vi "一体站流程自动启动.vi"(10 "二级进样":bool, 11 "参数":T1) -> ()   [LabVIEW 2016, in "PLC.lvlib"]
uses:
  PLC.lvlib
panel:
  out "s? t:f":enum16{"初始化", "采配水启动", "仪器操作", "反冲洗", "结束"}(ring)
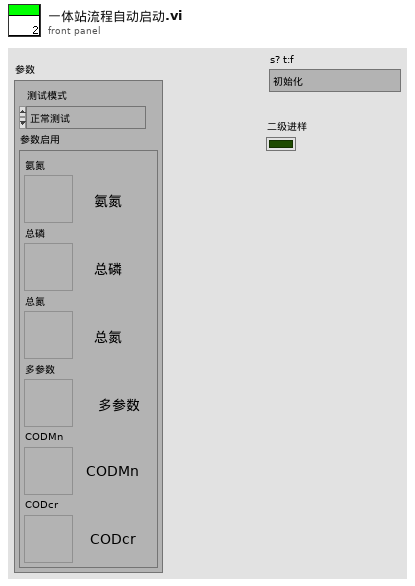
[diagram p1: front panel]
types:
  T1 = cluster{"测试模式":enum16{"正常测试", "集成干预"}, "参数启用":cluster{"氨氮":bool, "总磷":bool, "总氮":bool, "多参数":bool, "CODMn":bool, "CODcr":bool}}
  T2 = cluster{"命令":string, cluster{"starting address":u16, "holding register value":u16}}
  T3 = enum16{"启动测量", "标样核查", "零点核查", "跨度核查", "空白测试", "平行样测试", "加标回收", "空白校准", "标样校准", "初始化（清洗）", "停止测试", "仪器重启", "校时", "模式设置", "测量间隔设置"}
  T4 = cluster{"时间标识":timestamp, "设备":string, "日志信息":string, "流程参数":string}
  T5 = cluster{"测量模式":enum16{"水样测量", "标样核查", "零点核查", "跨度核查", "空白测试", "加标回收", "平行样", "校零", "校标"}}
  T6 = cluster{"时间标识":timestamp, "设备":string, "日志信息":string}
  T7 = enum16{"空闲", "水样测试", "标样核查", "零点核查", "跨度核查", "空白测试", "平行样测试", "加标回收", "空白校准", "标样校准", "初始化（清洗）"}
  T8 = cluster{"R0":i16, "R1":i16, "R2":i16, "R3":i16, "R4":i16, "R5":i16, "R6":i16, "R7":i16, "R8":i16, "R9":i16, "R10":i16, "R11":i16, "R12":i16, "R13":i16, "R14":i16, "R15":i16, "R16":i16, "R17":i16, "R18":i16, "R19":i16, "R20":i16, "R21":i16, "R22":i16, "R23":i16, "R24":i16, "R25":i16, "R26":i16, "R27":i16, "R28":i16, "R29":i16, "R30":i16, "R31":i16, "R32":i16, "R33":i16, "R34":i16, "R35":i16, "R36":i16, "R37":i16, "R38":i16, "R39":i16, "R40":i16, "R41":i16, "R42":i16, "R43":i16, "R44":i16, "R45":i16, "R46":i16, "R47":i16, "R48":i16, "R49":i16, "R50":i16, "R51":i16, "R52":i16, "R53":i16, "R54":i16, "R55":i16, "R56":i16}
  T9 = cluster{"R100":i16, "R101":i16, "R102":i16, "R103":i16, "R104":i16, "R105":i16, "R106":i16, "R107":i16, "R108":i16, "R109":i16, "R110":i16, "R111":i16, "R112":i16, "R113":i16, "R114":i16, "R115":i16, "R116":i16, "R117":i16, "R118":i16, "R119":i16, "R120":i16, "R121":i16, "R122":i16, "R123":i16}
  T10 = enum32{"Bad", "Idle", "Run top level", "Running"}
  T11 = cluster{"氨氮":bool, "总磷":bool, "总氮":bool, "多参数":bool, "CODMn":bool, "CODcr":bool}
  T12 = cluster{"时间标识":timestamp, "参数":string, "集成干预测试浓度值":dbl, "集成干预前测试时间":timestamp, "集成干预前测试浓度值":dbl}
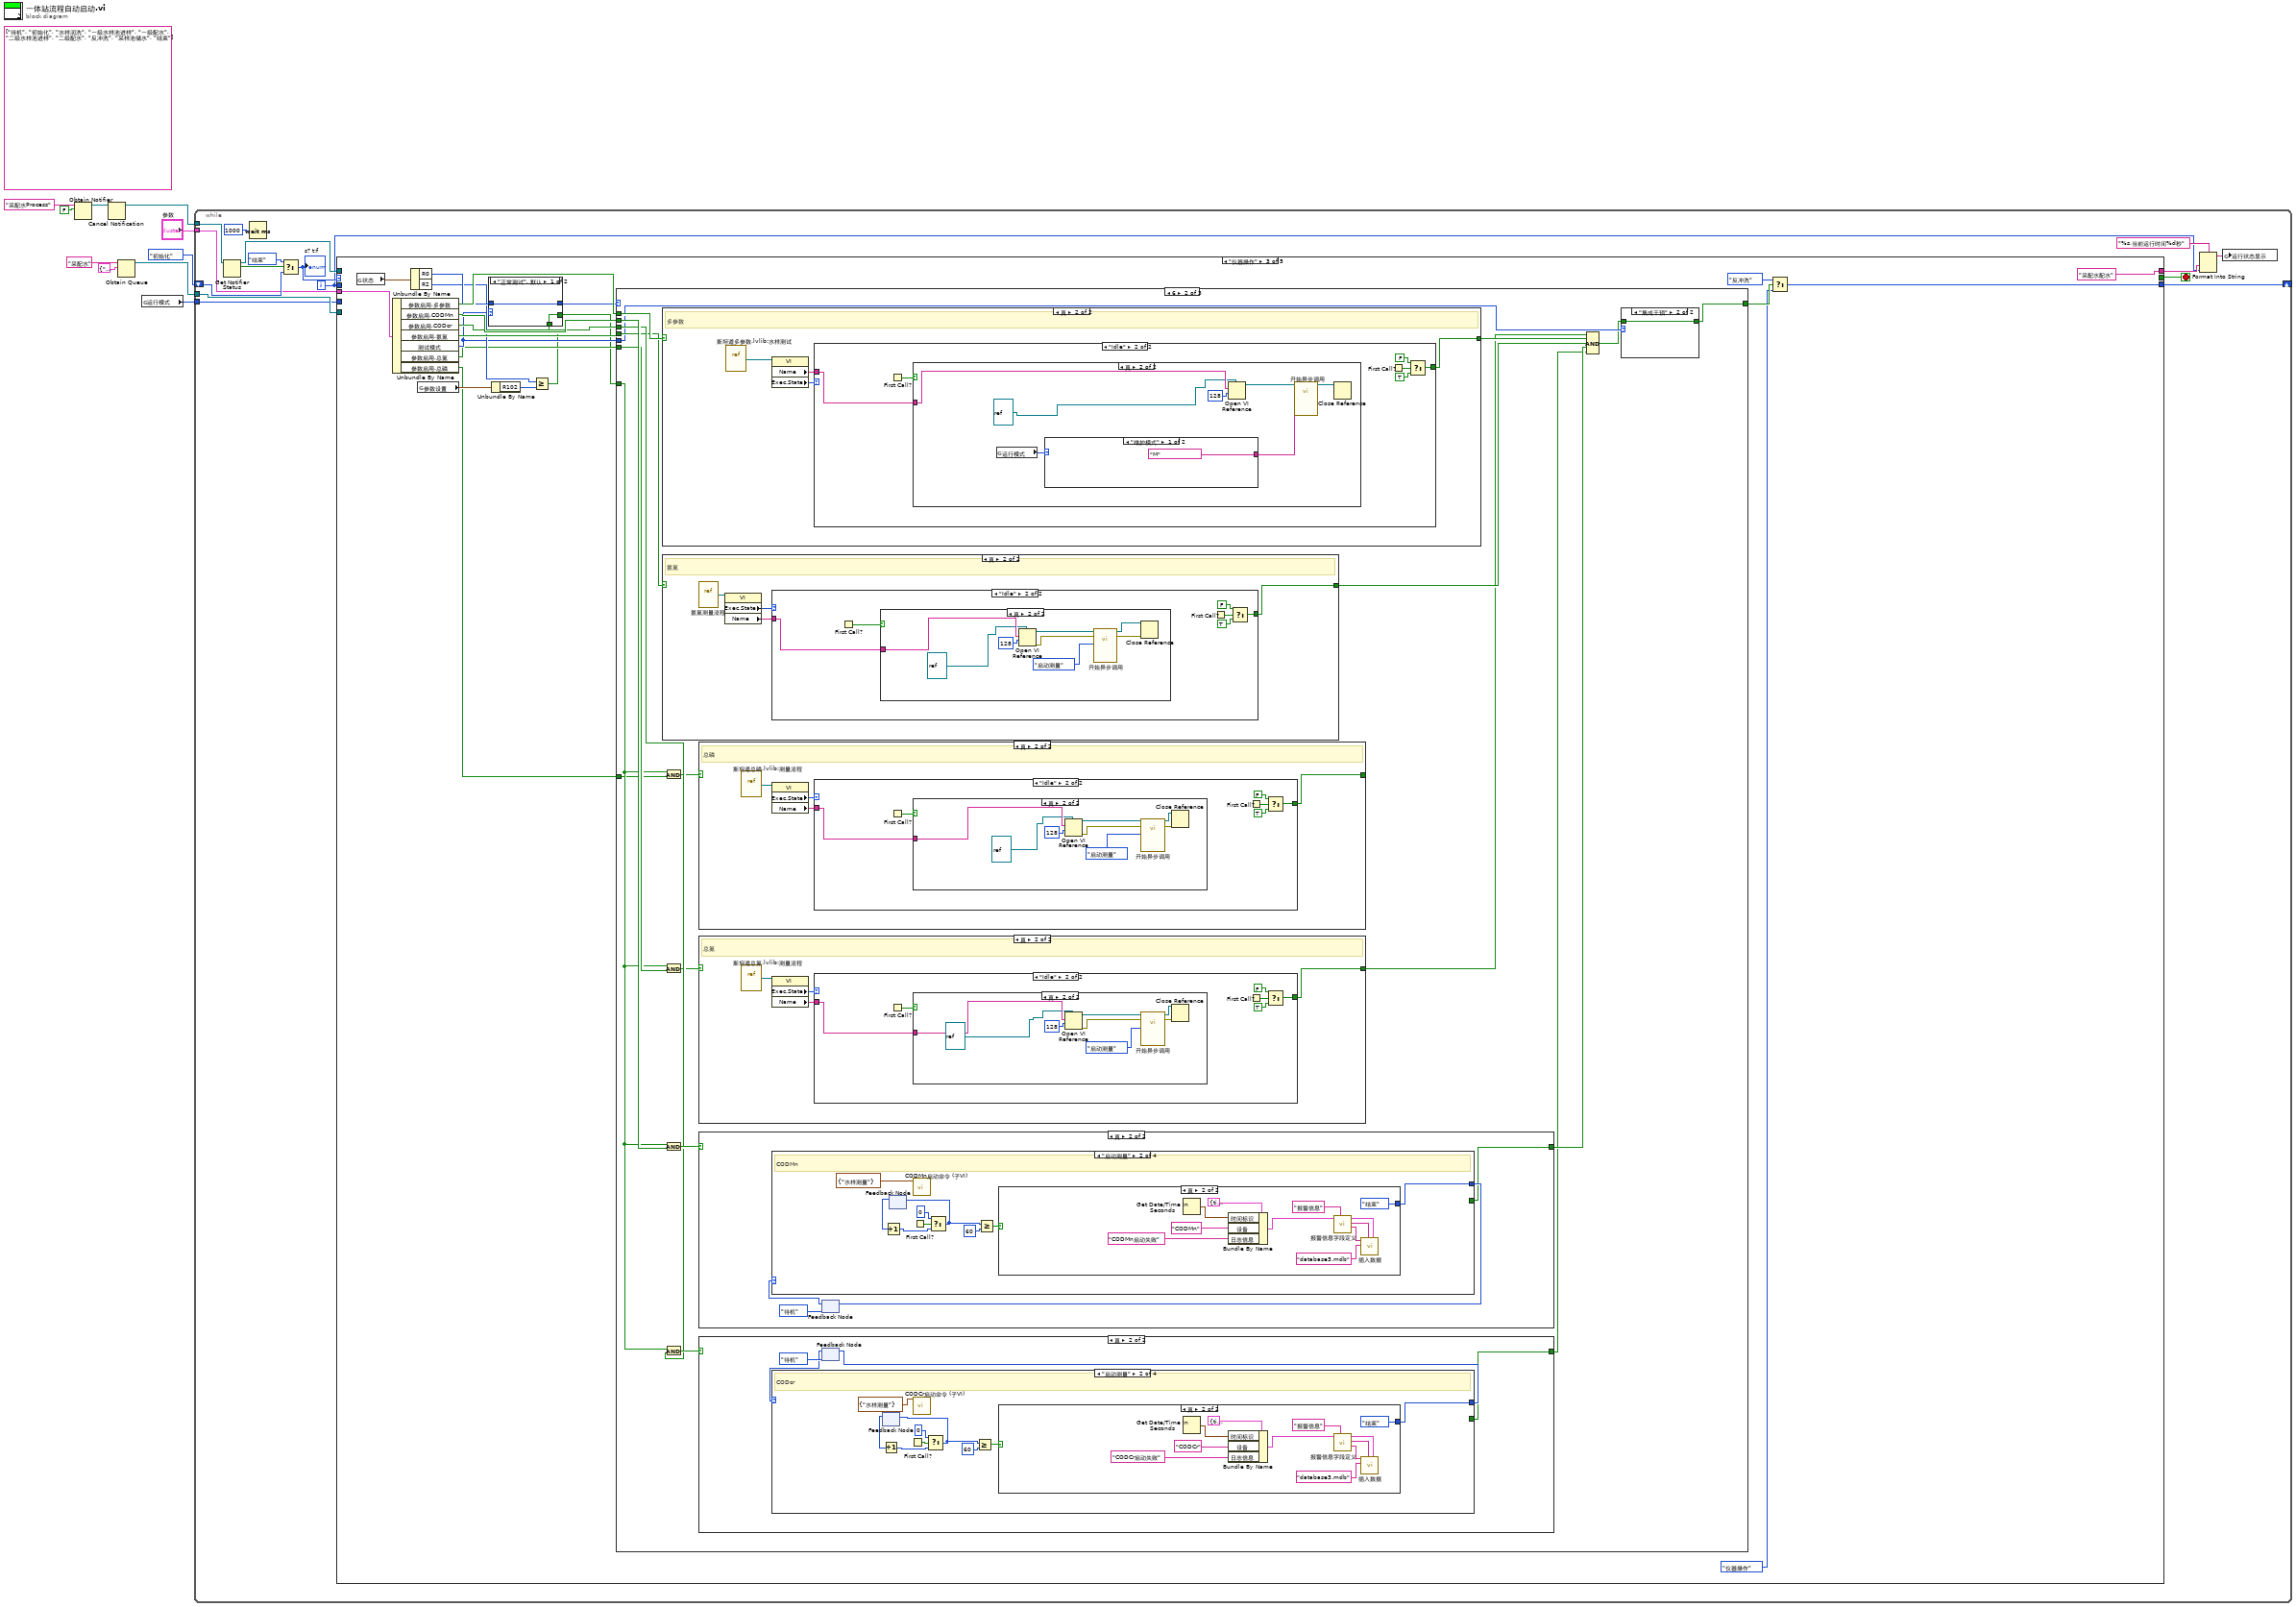
[diagram p0: block diagram]
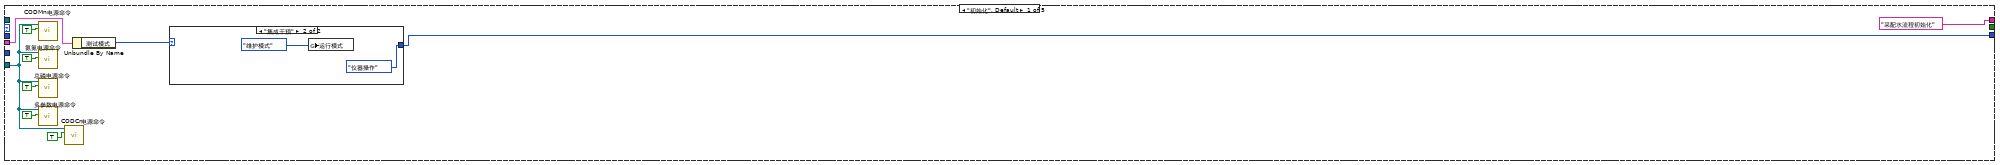
[diagram p2: hidden frame]
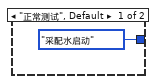
[diagram p3: hidden frame]
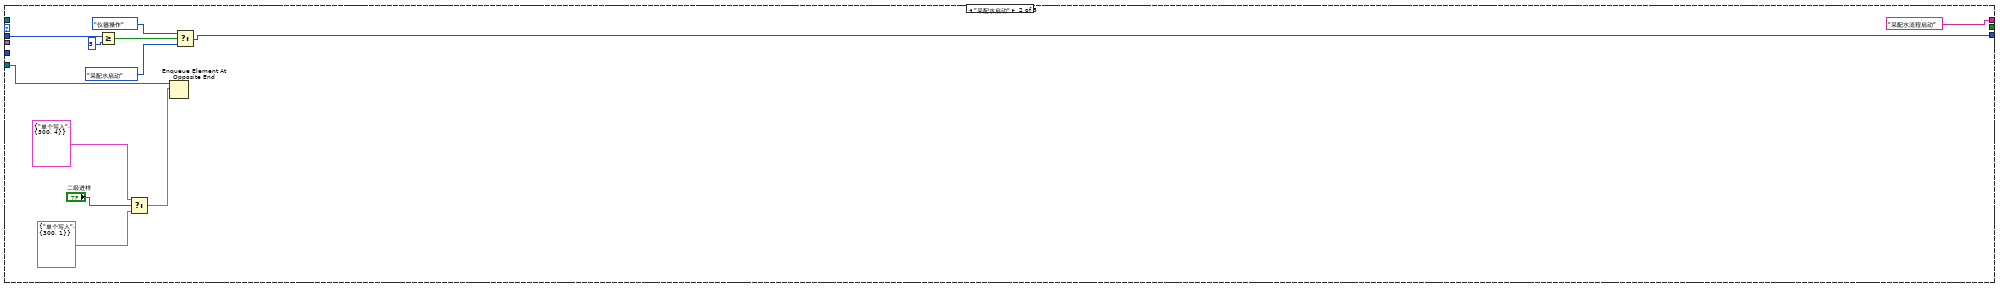
[diagram p4: hidden frame]
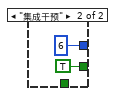
[diagram p5: hidden frame]
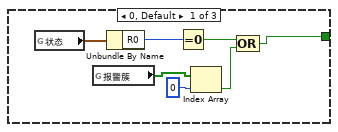
[diagram p6: hidden frame]
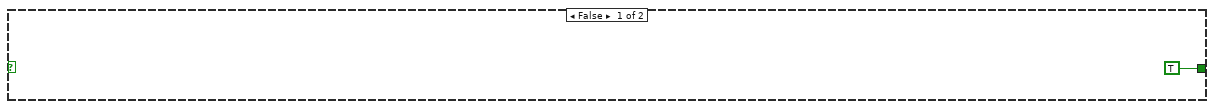
[diagram p7: hidden frame]
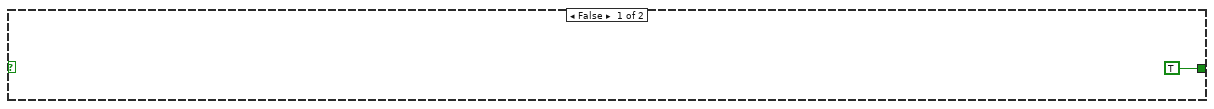
[diagram p10: hidden frame]
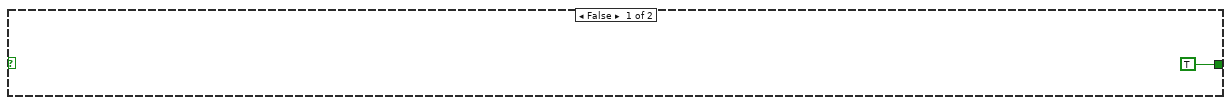
[diagram p14: hidden frame]
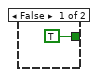
[diagram p17: hidden frame]
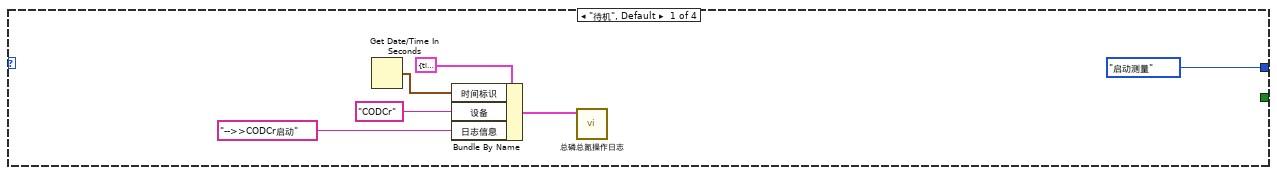
[diagram p18: hidden frame]
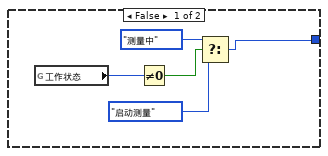
[diagram p19: hidden frame]
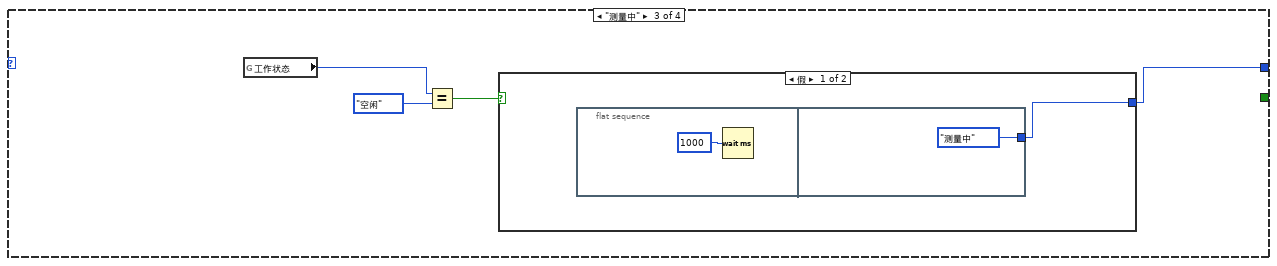
[diagram p20: hidden frame]
diagram:
  (unwired) string[][] [["待机"], ["初始化"], ["水样润洗"], ["一级水样池进样"], ["一级配水"], ["二级水样池进样"], ["二级配水"], ["反冲洗"], ["采样池储水"], ["结束"]] ("项名")
  n1 = Obtain Notifier(name (unnamed)="采配水Process" ("名称（未命名）"), notification data type=FALSE) -> (notifier out=w4:refnum<notifier>)  [unwired: 2 in, 2 out]
  n2 = Cancel Notification(0:w4) -> (8:w3:refnum<notifier>)  [unwired: 1 in, 2 out]
  n3 = Obtain Queue(name (unnamed)="采配水" ("名称（未命名）"), element data type=cluster{"命令":string, "数据":variant} {"命令"="", "数据"=variant}) -> (queue out=w7:refnum<queue>)  [unwired: 3 in, 2 out]
  n4 = global read "系统设置全局变量.vi" "运行模式"() -> (w1:enum16{"维护模式", "常规模式", "应急模式", "质控模式"})
  n5 = while {
    shift-right: [w23] -> _
    shift-left: enum16{"初始化", "采配水启动", "仪器操作", "反冲洗", "结束"}."初始化" ("枚举") -> [w19]
    tunnel: w7 -> [w26]
    tunnel: w3 -> [w22]
    tunnel: "参数" -> [w13]
    tunnel: w1 -> [w12]
    i -> [w11]
    stop <- w25 stop-if-true
    n6 = Get Notifier Status(notifier=w22) -> (notifier out=w14:refnum<notifier>, current notification=w21:bool)  [unwired: 1 in, 3 out]
    n7 = Wait (ms)(milliseconds to wait=u32 1000 ("等待时间（毫秒）")) -> ()  [unwired: 1 out]
    n8 = Select(t=enum16{"初始化", "采配水启动", "仪器操作", "反冲洗", "结束"}."结束" ("枚举"), s=w21, f=w19) -> (s? t:f=w18:enum16{"初始化", "采配水启动", "仪器操作", "反冲洗", "结束"})
    "s? t:f" <- w18
    n9 = case shown="\"仪器操作\"" w18 {
      tunnel: w26 -> [w31 w51 _ _ w456]
      tunnel: [_ _ _ _ TRUE] -> w25
      tunnel: [w30 w44 w67 w288 enum16{"初始化", "采配水启动", "仪器操作", "反冲洗", "结束"}."结束" ("枚举")] -> w23
      tunnel: ["采配水流程初始化" "采配水流程启动" "采配水配水" "等待测试完成" "采配水结束"] -> w15
      tunnel: w14 -> [_ _ _ _ w457]
      tunnel: w13 -> [w28 _ w70 w287 w453]
      tunnel: w12 -> [_ _ _ _ w452]
      tunnel: w11 -> [_ w49 _ _ _]
      frame "初始化", Default {
        n10 = call "CODMn电源命令.vi"("通电/断电"=TRUE, "队列"=w31) -> ()  [unwired: 9 in, 1 out]
        n11 = call "氨氮电源命令.vi"("通电/断电"=TRUE, "队列"=w31) -> ()  [unwired: 9 in, 1 out]
        n12 = call "总磷电源命令.vi"("通电/断电"=TRUE, "队列"=w31) -> ()  [unwired: 9 in, 1 out]
        n13 = call "多参数电源命令.vi"("通电/断电"=TRUE, "队列"=w31) -> ()  [unwired: 9 in, 1 out]
        n14 = call "CODCr电源命令.vi"("通电/断电"=TRUE, "队列"=w31) -> ()  [unwired: 9 in, 1 out]
        n15 = Unbundle By Name(w28) -> ("测试模式"=w27:enum16{"正常测试", "集成干预"})
        n16 = case shown="\"集成干预\"" w27 {
          tunnel: [enum16{"初始化", "采配水启动", "仪器操作", "反冲洗", "结束"}."采配水启动" ("枚举") enum16{"初始化", "采配水启动", "仪器操作", "反冲洗", "结束"}."仪器操作" ("枚举")] -> w30
          frame "正常测试", Default {
          }
          frame "集成干预" {
            n17 = global write "系统设置全局变量.vi" "运行模式"(enum16{"维护模式", "常规模式", "应急模式", "质控模式"}."维护模式" ("运行模式")) -> ()
          }
        }
      }
      frame "采配水启动" {
        n18 = Greater Or Equal?(x=w49, y=5) -> (x >= y?=w47:bool)
        n19 = Select(t=T2 {"命令"="单个写入", {"starting address"=300, "holding register value"=4}} ("元素"), s="二级进样", f=T2 {"命令"="单个写入", {"starting address"=300, "holding register value"=1}} ("元素")) -> (s? t:f=w40:T2)
        n20 = Enqueue Element At Opposite End(queue=w51, element=w40) -> ()  [unwired: 2 in, 3 out]
        n21 = Select(t=enum16{"初始化", "采配水启动", "仪器操作", "反冲洗", "结束"}."仪器操作" ("枚举"), s=w47, f=enum16{"初始化", "采配水启动", "仪器操作", "反冲洗", "结束"}."采配水启动" ("枚举")) -> (s? t:f=w44:enum16{"初始化", "采配水启动", "仪器操作", "反冲洗", "结束"})
      }
      frame "仪器操作" {
        n22 = global read "采配水全局变量.vi" "状态"() -> (w72:T8)
        n23 = Unbundle By Name(w70) -> ("参数启用.多参数"=w65:bool, "参数启用.CODMn"=w64:bool, "参数启用.CODcr"=w63:bool, "参数启用.氨氮"=w62:bool, "测试模式"=w56:enum16{"正常测试", "集成干预"}, "参数启用.总氮"=w55:bool, "参数启用.总磷"=w54:bool)
        n24 = Unbundle By Name(w72) -> ("R0"=w61:i16, "R2"=w57:i16)
        n25 = global read "采配水全局变量.vi" "参数设置"() -> (w58:T9)
        n26 = Unbundle By Name(w58) -> ("R102"=w59:i16)
        n27 = Greater Or Equal?(x=w57, y=w59) -> (x >= y?=w53:bool)
        n28 = case shown="\"正常测试\", 默认" w56 {
          tunnel: w61 -> [w74 _]
          tunnel: [w74 i16 6 ("R0")] -> w60
          tunnel: w53 -> [w73 _]
          tunnel: [w73 TRUE] -> w52
          frame "正常测试", Default {
          }
          frame "集成干预" {
          }
        }
        n29 = case shown="6" w60 {
          tunnel: [w78 w90 TRUE] -> w69
          tunnel: w65 -> [_ w102 _]
          tunnel: w64 -> [_ w101 _]
          tunnel: w63 -> [_ w98 _]
          tunnel: w62 -> [_ w97 _]
          tunnel: w52 -> [_ w86 _]
          tunnel: w56 -> [_ w92 _]
          tunnel: w55 -> [_ w89 _]
          tunnel: w54 -> [_ w85 _]
          frame 0, Default {
            n30 = global read "采配水全局变量.vi" "状态"() -> (w81:T8)
            n31 = global read "采配水全局变量.vi" "报警簇"() -> (w82:bool[])
            n32 = Unbundle By Name(w81) -> ("R0"=w80:i16)
            n33 = Equal To 0?(x=w80) -> (x = 0?=w83:bool)
            n34 = Index Array(array=w82, index=0 ("索引")) -> (element=w77:bool)
            n35 = Compound Arithmetic op=OR ("复合运算")(w83, w77) -> (w78:bool)
          }
          frame 6 {
            n36 = case shown="真" w102 {
              tunnel: [TRUE ("t") w268] -> w96
              frame False {
              }
              frame True {
                # "多参数"
                n37 = vi-ref "斯坦道多参数.lvlib:水样测试.vi"() -> (w266:refnum<vi>)
                n38 = property class="VI"(reference=w266) -> ("Name"=w265:string, "Exec.State"=w267:T10)  [unwired: 1 in, 2 out]
                n39 = case shown="\"Idle\"" w267 {
                  tunnel: w265 -> [_ w274]
                  tunnel: [_ w269] -> w268
                  frame "Bad", Default {
                  }
                  frame "Idle" {
                    n40 = First Call?() -> (First Call?: T/F=w273:bool)
                    n41 = case shown="真" w273 {
                      tunnel: w274 -> [_ w280]
                      frame False {
                      }
                      frame True {
                        n42 = global read "系统设置全局变量.vi" "运行模式"() -> (w277:enum16{"维护模式", "常规模式", "应急模式", "质控模式"})
                        n43 = case shown="\"维护模式\"" w277 {
                          tunnel: ["M" ("数据标记表") "N" ("数据标记表")] -> w276
                          frame "维护模式" {
                          }
                          frame "常规模式", Default {
                          }
                        }
                        n44 = Open VI Reference(type specifier VI Refnum (for type only)=refnum<vi> refnum, vi path=w280, options=128 ("选项")) -> (vi reference=w279:refnum<vi>)  [unwired: 3 in, 1 out]
                        n45 = call-by-ref "开始异步调用"(reference=w279, "数据标记表"=w276) -> (reference out=w278:refnum<vi>)  [unwired: 12 in, 1 out]
                        n46 = Close Reference(reference=w278) -> ()  [unwired: 1 in, 1 out]
                      }
                    }
                    n47 = First Call?() -> (First Call?: T/F=w272:bool)
                    n48 = Select(t=FALSE, s=w272, f=TRUE) -> (s? t:f=w269:bool)
                  }
                }
              }
            }
            n49 = case "条件结构" shown="真" w97 {
              tunnel: [TRUE ("t") w143] -> w95
              frame False {
              }
              frame True {
                # "氨氮"
                n50 = vi-ref "氨氮测量流程.vi"() -> (w146:refnum<vi>)
                n51 = property class="VI"(reference=w146) -> ("Exec.State"=w145:T10, "Name"=w144:string)  [unwired: 1 in, 2 out]
                n52 = case shown="\"Idle\"" w145 {
                  tunnel: w144 -> [_ w152]
                  tunnel: [_ w147] -> w143
                  frame "Bad", Default {
                  }
                  frame "Idle" {
                    n53 = First Call?() -> (First Call?: T/F=w151:bool)
                    n54 = case shown="真" w151 {
                      tunnel: w152 -> [_ w157]
                      frame False {
                      }
                      frame True {
                        n55 = Open VI Reference(type specifier VI Refnum (for type only)=refnum<vi> refnum, vi path=w157, options=128 ("选项")) -> (vi reference=w155:refnum<vi>, error out=w158:errorcluster)  [unwired: 3 in]
                        n56 = call-by-ref "开始异步调用"(reference=w155, error in=w158, "控制命令"=T3."启动测量") -> (reference out=w159:refnum<vi>, error out=w160:errorcluster)  [unwired: 11 in]
                        n57 = Close Reference(reference=w159, error in (no error)=w160) -> ()  [unwired: 1 out]
                      }
                    }
                    n58 = First Call?() -> (First Call?: T/F=w150:bool)
                    n59 = Select(t=FALSE, s=w150, f=TRUE) -> (s? t:f=w147:bool)
                  }
                }
              }
            }
            n60 = And(x=w86, y=w85) -> (x .and. y?=w84:bool)
            n61 = And(x=w86, y=w89) -> (x .and. y?=w88:bool)
            n62 = And(x=w86, y=w101) -> (x .and. y?=w100:bool)
            n63 = And(x=w86, y=w98) -> (x .and. y?=w99:bool)
            n64 = case "条件结构" shown="真" w84 {
              tunnel: [TRUE ("t") w104] -> _
              frame False {
              }
              frame True {
                # "总磷"
                n65 = vi-ref "斯坦道总磷.lvlib:测量流程.vi"() -> (w107:refnum<vi>)
                n66 = property class="VI"(reference=w107) -> ("Exec.State"=w106:T10, "Name"=w105:string)  [unwired: 1 in, 2 out]
                n67 = case shown="\"Idle\"" w106 {
                  tunnel: w105 -> [_ w113]
                  tunnel: [_ w108] -> w104
                  frame "Bad", Default {
                  }
                  frame "Idle" {
                    n68 = First Call?() -> (First Call?: T/F=w112:bool)
                    n69 = case shown="真" w112 {
                      tunnel: w113 -> [_ w118]
                      frame False {
                      }
                      frame True {
                        n70 = Open VI Reference(type specifier VI Refnum (for type only)=refnum<vi> refnum, vi path=w118, options=128 ("选项")) -> (vi reference=w116:refnum<vi>, error out=w119:errorcluster)  [unwired: 3 in]
                        n71 = call-by-ref "开始异步调用"(reference=w116, error in=w119, "控制命令"=T3."启动测量") -> (reference out=w120:refnum<vi>, error out=w121:errorcluster)  [unwired: 11 in]
                        n72 = Close Reference(reference=w120, error in (no error)=w121) -> ()  [unwired: 1 out]
                      }
                    }
                    n73 = First Call?() -> (First Call?: T/F=w111:bool)
                    n74 = Select(t=FALSE, s=w111, f=TRUE) -> (s? t:f=w108:bool)
                  }
                }
              }
            }
            n75 = case "条件结构" shown="真" w88 {
              tunnel: [TRUE ("t") w123] -> w87
              frame False {
              }
              frame True {
                # "总氮"
                n76 = vi-ref "斯坦道总氮.lvlib:测量流程.vi"() -> (w126:refnum<vi>)
                n77 = property class="VI"(reference=w126) -> ("Exec.State"=w125:T10, "Name"=w124:string)  [unwired: 1 in, 2 out]
                n78 = case shown="\"Idle\"" w125 {
                  tunnel: w124 -> [_ w132]
                  tunnel: [_ w127] -> w123
                  frame "Bad", Default {
                  }
                  frame "Idle" {
                    n79 = First Call?() -> (First Call?: T/F=w131:bool)
                    n80 = case shown="真" w131 {
                      tunnel: w132 -> [_ w137]
                      frame False {
                      }
                      frame True {
                        n81 = Open VI Reference(type specifier VI Refnum (for type only)=refnum<vi> refnum, vi path=w137, options=128 ("选项")) -> (vi reference=w135:refnum<vi>, error out=w138:errorcluster)  [unwired: 3 in]
                        n82 = call-by-ref "开始异步调用"(reference=w135, error in=w138, "控制命令"=T3."启动测量") -> (reference out=w139:refnum<vi>, error out=w140:errorcluster)  [unwired: 11 in]
                        n83 = Close Reference(reference=w139, error in (no error)=w140) -> ()  [unwired: 1 out]
                      }
                    }
                    n84 = First Call?() -> (First Call?: T/F=w130:bool)
                    n85 = Select(t=FALSE, s=w130, f=TRUE) -> (s? t:f=w127:bool)
                  }
                }
              }
            }
            n86 = case shown="真" w100 {
              tunnel: [TRUE w214] -> w94
              frame False {
              }
              frame True {
                n87 = feedback #1(enum16{"待机", "启动测量", "测量中", "结束"}."待机") -> (w216:enum16{"待机", "启动测量", "测量中", "结束"})
                n88 = case shown="\"启动测量\"" w216 {
                  tunnel: [enum16{"待机", "启动测量", "测量中", "结束"}."启动测量" w232 w251 enum16{"待机", "启动测量", "测量中", "结束"}."结束"] -> w215
                  tunnel: [_ _ _ TRUE] -> w214
                  frame "待机", Default {
                    n89 = Get Date/Time In Seconds() -> (seconds since 1Jan1904=w222:timestamp)
                    n90 = Bundle By Name(cluster=T4 {"时间标识"=timestamp(0 s since 1904-01-01), "设备"="", "日志信息"="", "流程参数"=""} ("data in"), "时间标识"=w222, "设备"="CODMn", "日志信息"="-->>CODMn启动") -> (w218:T4)
                    n91 = call "总磷总氮操作日志.vi"("data in"=w218) -> ()  [unwired: 11 in]
                  }
                  frame "启动测量" {
                    # "CODMn"
                    n92 = feedback #2() -> (w228:i32)  [unwired: 1 in]
                    n93 = Increment(x=w228) -> (x+1=w229:i32)
                    n94 = First Call?() -> (First Call?: T/F=w227:bool)
                    n95 = call "CODMn启动命令 (子VI).vi"("启动测量模式"=T5 {"测量模式"=enum."水样测量"}) -> ()  [unwired: 11 in]
                    n96 = Select(t=0, s=w227, f=w229) -> (s? t:f=w230:i32)
                    n97 = feedback-in #2(w230) -> ()
                    n98 = Greater Or Equal?(x=w230, y=60) -> (x >= y?=w225:bool)
                    n99 = case shown="真" w225 {
                      tunnel: [w234 enum16{"待机", "启动测量", "测量中", "结束"}."结束"] -> w232
                      frame False {
                        n100 = global read "运行时序全局变量.vi" "多列列表框"() -> (w233:i32)
                        n101 = Not Equal To 0?(x=w233) -> (x != 0?=w235:bool)
                        n102 = Select(t=enum16{"待机", "启动测量", "测量中", "结束"}."测量中", s=w235, f=enum16{"待机", "启动测量", "测量中", "结束"}."启动测量") -> (s? t:f=w234:enum16{"待机", "启动测量", "测量中", "结束"})
                      }
                      frame True {
                        n103 = Get Date/Time In Seconds() -> (seconds since 1Jan1904=w244:timestamp)
                        n104 = Bundle By Name(cluster=T6 {"时间标识"=timestamp(0 s since 1904-01-01), "设备"="", "日志信息"=""} ("data in"), "时间标识"=w244, "设备"="CODMn", "日志信息"="CODMn启动失败") -> (w238:T6)
                        n105 = call "报警信息字段定义.vi"("table输入"="报警信息", "data in"=w238) -> ("table输出"=w241:string, "columns"=w242:string[], "data out"=w243:T6)  [unwired: 7 in]
                        n106 = call "插入数据.vi"("data"=w243, "columns"=w242, "database"="database3.mdb", "table"=w241) -> ()  [unwired: 7 in, 1 out]
                      }
                    }
                  }
                  frame "测量中" {
                    n107 = global read "运行时序全局变量.vi" "多列列表框"() -> (w250:i32)
                    n108 = Equal To 0?(x=w250) -> (x = 0?=w249:bool)
                    n109 = case shown="假" w249 {
                      tunnel: [w252 enum16{"待机", "启动测量", "测量中", "结束"}."结束"] -> w251
                      frame False {
                        n110 = flat-sequence {
                          tunnel: [enum16{"待机", "启动测量", "测量中", "结束"}."测量中"] -> w252
                          frame #0 {
                            n111 = Wait (ms)(milliseconds to wait=u32 1000 ("等待时间（毫秒）")) -> ()  [unwired: 1 out]
                          }
                          frame #1 {
                          }
                        }
                      }
                      frame True {
                      }
                    }
                  }
                  frame "结束" {
                    n112 = First Call?() -> (First Call?: T/F=w256:bool)
                    n113 = case shown="真" w256 {
                      frame False {
                      }
                      frame True {
                        n114 = Get Date/Time In Seconds() -> (seconds since 1Jan1904=w263:timestamp)
                        n115 = Bundle By Name(cluster=T4 {"时间标识"=timestamp(0 s since 1904-01-01), "设备"="", "日志信息"="", "流程参数"=""} ("data in"), "时间标识"=w263, "设备"="CODMn", "日志信息"="-->>CODMn停止") -> (w259:T4)
                        n116 = call "总磷总氮操作日志.vi"("data in"=w259) -> ()  [unwired: 11 in]
                      }
                    }
                  }
                }
                n117 = feedback-in #1(w215) -> ()
              }
            }
            n118 = case shown="真" w99 {
              tunnel: [TRUE w162] -> w93
              frame False {
              }
              frame True {
                n119 = feedback #3(enum16{"待机", "启动测量", "测量中", "结束"}."待机") -> (w164:enum16{"待机", "启动测量", "测量中", "结束"})
                n120 = case shown="\"启动测量\"" w164 {
                  tunnel: [enum16{"待机", "启动测量", "测量中", "结束"}."启动测量" w180 w200 enum16{"待机", "启动测量", "测量中", "结束"}."结束"] -> w163
                  tunnel: [_ _ _ TRUE] -> w162
                  frame "待机", Default {
                    n121 = Get Date/Time In Seconds() -> (seconds since 1Jan1904=w170:timestamp)
                    n122 = Bundle By Name(cluster=T4 {"时间标识"=timestamp(0 s since 1904-01-01), "设备"="", "日志信息"="", "流程参数"=""} ("data in"), "时间标识"=w170, "设备"="CODCr", "日志信息"="-->>CODCr启动") -> (w166:T4)
                    n123 = call "总磷总氮操作日志.vi"("data in"=w166) -> ()  [unwired: 11 in]
                  }
                  frame "启动测量" {
                    # "CODcr"
                    n124 = feedback #4() -> (w176:i32)  [unwired: 1 in]
                    n125 = Increment(x=w176) -> (x+1=w177:i32)
                    n126 = First Call?() -> (First Call?: T/F=w175:bool)
                    n127 = call "CODCr启动命令 (子VI).vi"("启动测量模式"=T5 {"测量模式"=enum."水样测量"}) -> ()  [unwired: 11 in]
                    n128 = Select(t=0, s=w175, f=w177) -> (s? t:f=w178:i32)
                    n129 = feedback-in #4(w178) -> ()
                    n130 = Greater Or Equal?(x=w178, y=60) -> (x >= y?=w173:bool)
                    n131 = case shown="真" w173 {
                      tunnel: [w181 enum16{"待机", "启动测量", "测量中", "结束"}."结束"] -> w180
                      frame False {
                        n132 = global read "CODcr全局变量.vi" "工作状态"() -> (w182:T7)
                        n133 = Not Equal To 0?(x=w182) -> (x != 0?=w183:bool)
                        n134 = Select(t=enum16{"待机", "启动测量", "测量中", "结束"}."测量中", s=w183, f=enum16{"待机", "启动测量", "测量中", "结束"}."启动测量") -> (s? t:f=w181:enum16{"待机", "启动测量", "测量中", "结束"})
                      }
                      frame True {
                        n135 = Get Date/Time In Seconds() -> (seconds since 1Jan1904=w192:timestamp)
                        n136 = Bundle By Name(cluster=T6 {"时间标识"=timestamp(0 s since 1904-01-01), "设备"="", "日志信息"=""} ("data in"), "时间标识"=w192, "设备"="CODCr", "日志信息"="CODCr启动失败") -> (w186:T6)
                        n137 = call "报警信息字段定义.vi"("table输入"="报警信息", "data in"=w186) -> ("table输出"=w189:string, "columns"=w190:string[], "data out"=w191:T6)  [unwired: 7 in]
                        n138 = call "插入数据.vi"("data"=w191, "columns"=w190, "database"="database3.mdb", "table"=w189) -> ()  [unwired: 7 in, 1 out]
                      }
                    }
                  }
                  frame "测量中" {
                    n139 = global read "CODcr全局变量.vi" "工作状态"() -> (w199:T7)
                    n140 = Equal?(x=w199, y=T7."空闲" ("工作状态")) -> (x = y?=w198:bool)
                    n141 = case shown="假" w198 {
                      tunnel: [w201 enum16{"待机", "启动测量", "测量中", "结束"}."结束"] -> w200
                      frame False {
                        n142 = flat-sequence {
                          tunnel: [enum16{"待机", "启动测量", "测量中", "结束"}."测量中"] -> w201
                          frame #0 {
                            n143 = Wait (ms)(milliseconds to wait=u32 1000 ("等待时间（毫秒）")) -> ()  [unwired: 1 out]
                          }
                          frame #1 {
                          }
                        }
                      }
                      frame True {
                      }
                    }
                  }
                  frame "结束" {
                    n144 = First Call?() -> (First Call?: T/F=w205:bool)
                    n145 = case shown="真" w205 {
                      frame False {
                      }
                      frame True {
                        n146 = Get Date/Time In Seconds() -> (seconds since 1Jan1904=w212:timestamp)
                        n147 = Bundle By Name(cluster=T4 {"时间标识"=timestamp(0 s since 1904-01-01), "设备"="", "日志信息"="", "流程参数"=""} ("data in"), "时间标识"=w212, "设备"="CODCr", "日志信息"="-->>CODCr停止") -> (w208:T4)
                        n148 = call "总磷总氮操作日志.vi"("data in"=w208) -> ()  [unwired: 11 in]
                      }
                    }
                  }
                }
                n149 = feedback-in #3(w163) -> ()
              }
            }
            n150 = Compound Arithmetic op=AND ("复合运算")(w87, w96, w95, w94, w93) -> (w91:bool)
            n151 = case shown="\"集成干预\"" w92 {
              tunnel: w91 -> [_ w141]
              tunnel: [_ w141] -> w90
              frame "正常测试", Default {
              }
              frame "集成干预" {
              }
            }
          }
          frame 7..9 {
          }
        }
        n152 = Select(t=enum16{"初始化", "采配水启动", "仪器操作", "反冲洗", "结束"}."反冲洗" ("枚举"), s=w69, f=enum16{"初始化", "采配水启动", "仪器操作", "反冲洗", "结束"}."仪器操作" ("枚举")) -> (s? t:f=w67:enum16{"初始化", "采配水启动", "仪器操作", "反冲洗", "结束"})
      }
      frame "反冲洗" {
        n153 = First Call?() -> (First Call?: T/F=w285:bool)
        n154 = case shown="真" w285 {
          tunnel: w287 -> [_ w296]
          frame False {
          }
          frame True {
            n155 = Unbundle By Name(w296) -> ("测试模式"=w295:enum16{"正常测试", "集成干预"}, "参数启用"=w294:T11)
            n156 = case shown="\"正常测试\", 默认" w295 {
              tunnel: w294 -> [w299 w385]
              frame "正常测试", Default {
                n157 = global read "系统设置全局变量.vi" "运行模式"() -> (w297:enum16{"维护模式", "常规模式", "应急模式", "质控模式"})
                n158 = global read "采配水全局变量.vi" "报警簇"() -> (w304:bool[])
                n159 = case shown="\"维护模式\"" w297 {
                  tunnel: ["M" ("table") "N" ("table")] -> w298
                  frame "维护模式" {
                  }
                  frame "常规模式", Default {
                  }
                }
                n160 = Index Array(array=w304, index #1=0 ("索引"), index #2=11 ("索引")) -> (element #1=w301:bool, element #2=w300:bool)
                n161 = case shown="真" w301 {
                  tunnel: w300 -> [w310 _]
                  tunnel: w299 -> [w309 w324]
                  tunnel: w298 -> [w307 w318]
                  frame False {
                    n162 = Unbundle By Name(w309) -> ("氨氮"=w308:bool)
                    n163 = case shown="真" w310 {
                      tunnel: w308 -> [_ w312]
                      tunnel: w307 -> [_ w311]
                      frame False {
                      }
                      frame True {
                        n164 = case shown="真" w312 {
                          tunnel: w311 -> [_ w313]
                          tunnel: [_ w314] -> _
                          frame False {
                          }
                          frame True {
                            n165 = call "取水点无水样数据存储.vi"("数据标识"="lw", "数据类型"=w313, "table"="氨氮") -> ("error out"=w314:errorcluster)  [unwired: 8 in]
                          }
                        }
                      }
                    }
                  }
                  frame True {
                    n166 = Unbundle By Name(w324) -> ("氨氮"=w323:bool, "CODMn"=w322:bool, "CODcr"=w321:bool, "多参数"=w320:bool, "总氮"=w319:bool, "总磷"=w317:bool)
                    n167 = case shown="真" w323 {
                      tunnel: w318 -> [_ w375]
                      tunnel: [_ w376] -> _
                      frame False {
                      }
                      frame True {
                        n168 = call "取水点无水样数据存储.vi"("数据标识"="Z", "数据类型"=w375, "table"="氨氮") -> ("error out"=w376:errorcluster)  [unwired: 8 in]
                      }
                    }
                    n169 = case shown="真" w319 {
                      tunnel: w318 -> [_ w328]
                      frame False {
                      }
                      frame True {
                        n170 = call "取水点无水样数据存储.vi"("数据标识"="Z", "数据类型"=w328, "table"="总氮") -> ()  [unwired: 8 in, 1 out]
                      }
                    }
                    n171 = case shown="真" w322 {
                      tunnel: w318 -> [_ w372]
                      tunnel: [_ w371] -> _
                      frame False {
                      }
                      frame True {
                        n172 = call "取水点无水样数据存储.vi"("数据标识"="Z", "数据类型"=w372, "table"="CODMn") -> ("error out"=w371:errorcluster)  [unwired: 8 in]
                      }
                    }
                    n173 = case shown="真" w321 {
                      tunnel: w318 -> [_ w368]
                      tunnel: [_ w367] -> _
                      frame False {
                      }
                      frame True {
                        n174 = call "取水点无水样数据存储.vi"("数据标识"="Z", "数据类型"=w368, "table"="CODCr") -> ("error out"=w367:errorcluster)  [unwired: 8 in]
                      }
                    }
                    n175 = case shown="真" w320 {
                      tunnel: w318 -> [_ w338]
                      frame False {
                      }
                      frame True {
                        n176 = global read "断电保存变量.vi" "Cond"() -> (w332:bool)
                        n177 = global read "断电保存变量.vi" "Turb"() -> (w333:bool)
                        n178 = global read "断电保存变量.vi" "DO"() -> (w334:bool)
                        n179 = global read "断电保存变量.vi" "pH"() -> (w335:bool)
                        n180 = global read "断电保存变量.vi" "Temp"() -> (w336:bool)
                        n181 = case shown="真" w335 {
                          tunnel: w338 -> [_ w360]
                          tunnel: [_ w359] -> _
                          frame False {
                          }
                          frame True {
                            n182 = call "取水点无水样数据存储.vi"("数据标识"="Z", "数据类型"=w360, "table"="pH") -> ("error out"=w359:errorcluster)  [unwired: 8 in]
                          }
                        }
                        n183 = case shown="真" w334 {
                          tunnel: w338 -> [_ w356]
                          tunnel: [_ w355] -> _
                          frame False {
                          }
                          frame True {
                            n184 = call "取水点无水样数据存储.vi"("数据标识"="Z", "数据类型"=w356, "table"="DO") -> ("error out"=w355:errorcluster)  [unwired: 8 in]
                          }
                        }
                        n185 = case shown="真" w333 {
                          tunnel: w338 -> [_ w348]
                          tunnel: [_ w347] -> _
                          frame False {
                          }
                          frame True {
                            n186 = call "取水点无水样数据存储.vi"("数据标识"="Z", "数据类型"=w348, "table"="浊度") -> ("error out"=w347:errorcluster)  [unwired: 8 in]
                          }
                        }
                        n187 = case shown="真" w332 {
                          tunnel: w338 -> [_ w352]
                          tunnel: [_ w351] -> _
                          frame False {
                          }
                          frame True {
                            n188 = call "取水点无水样数据存储.vi"("数据标识"="Z", "数据类型"=w352, "table"="比电导率") -> ("error out"=w351:errorcluster)  [unwired: 8 in]
                          }
                        }
                        n189 = case shown="真" FALSE {
                          tunnel: w338 -> [_ w340]
                          tunnel: [_ w339] -> _
                          frame False {
                          }
                          frame True {
                            n190 = call "取水点无水样数据存储.vi"("数据标识"="Z", "数据类型"=w340, "table"="藻密度") -> ("error out"=w339:errorcluster)  [unwired: 8 in]
                          }
                        }
                        n191 = global read "断电保存变量.vi" "叶绿素a启用"() -> (w331:bool)
                        n192 = case shown="真" w336 {
                          tunnel: w338 -> [_ w364]
                          tunnel: [_ w363] -> _
                          frame False {
                          }
                          frame True {
                            n193 = call "取水点无水样数据存储.vi"("数据标识"="Z", "数据类型"=w364, "table"="水温") -> ("error out"=w363:errorcluster)  [unwired: 8 in]
                          }
                        }
                        n194 = case shown="真" w331 {
                          tunnel: w338 -> [_ w344]
                          tunnel: [_ w343] -> _
                          frame False {
                          }
                          frame True {
                            n195 = call "取水点无水样数据存储.vi"("数据标识"="Z", "数据类型"=w344, "table"="叶绿素") -> ("error out"=w343:errorcluster)  [unwired: 8 in]
                          }
                        }
                      }
                    }
                    n196 = case shown="真" w317 {
                      tunnel: [_ w325] -> _
                      frame False {
                      }
                      frame True {
                        n197 = call "取水点无水样数据存储.vi"("数据标识"="Z", "table"="总磷") -> ("error out"=w325:errorcluster)  [unwired: 9 in]
                      }
                    }
                  }
                }
              }
              frame "集成干预" {
                n198 = Unbundle By Name(w385) -> ("总磷"=w379:bool, "总氮"=w380:bool, "氨氮"=w384:bool, "CODMn"=w383:bool, "CODcr"=w382:bool, "多参数"=w381:bool)
                n199 = case shown="真" w379 {
                  frame False {
                  }
                  frame True {
                    n200 = call "获取最近两组水样测试数据.vi"("table"="总磷") -> ("error out"=w391:errorcluster, "存储变量"=w390:T12)  [unwired: 9 in]
                    n201 = call "集成干预测试数据存储.vi"("error in (no error)"=w391, "存储变量"=w390) -> ()  [unwired: 9 in, 1 out]
                  }
                }
                n202 = case shown="真" w380 {
                  frame False {
                  }
                  frame True {
                    n203 = call "获取最近两组水样测试数据.vi"("table"="总氮") -> ("error out"=w388:errorcluster, "存储变量"=w387:T12)  [unwired: 9 in]
                    n204 = call "集成干预测试数据存储.vi"("error in (no error)"=w388, "存储变量"=w387) -> ()  [unwired: 9 in, 1 out]
                  }
                }
                n205 = case shown="真" w384 {
                  frame False {
                  }
                  frame True {
                    n206 = call "获取最近两组水样测试数据.vi"("table"="氨氮") -> ("error out"=w449:errorcluster, "存储变量"=w450:T12)  [unwired: 9 in]
                    n207 = call "集成干预测试数据存储.vi"("error in (no error)"=w449, "存储变量"=w450) -> ("error out"=w445:errorcluster)  [unwired: 9 in]
                    n208 = call "获取最近两组水样测试数据.vi"("error in (no error)"=w445, "table"="总磷") -> ("error out"=w448:errorcluster, "存储变量"=w447:T12)  [unwired: 8 in]
                    n209 = call "集成干预测试数据存储.vi"("error in (no error)"=w448, "存储变量"=w447) -> ()  [unwired: 9 in, 1 out]
                  }
                }
                n210 = case shown="真" w383 {
                  frame False {
                  }
                  frame True {
                    n211 = call "获取最近两组水样测试数据.vi"("table"="CODMn") -> ("error out"=w442:errorcluster, "存储变量"=w443:T12)  [unwired: 9 in]
                    n212 = call "集成干预测试数据存储.vi"("error in (no error)"=w442, "存储变量"=w443) -> ()  [unwired: 9 in, 1 out]
                  }
                }
                n213 = case shown="真" w382 {
                  frame False {
                  }
                  frame True {
                    n214 = call "获取最近两组水样测试数据.vi"("table"="CODCr") -> ("error out"=w439:errorcluster, "存储变量"=w440:T12)  [unwired: 9 in]
                    n215 = call "集成干预测试数据存储.vi"("error in (no error)"=w439, "存储变量"=w440) -> ()  [unwired: 9 in, 1 out]
                  }
                }
                n216 = case shown="真" w381 {
                  frame False {
                  }
                  frame True {
                    n217 = global read "断电保存变量.vi" "Temp"() -> (w398:bool)
                    n218 = case shown="真" w398 {
                      tunnel: [_ w435] -> w404
                      frame False {
                      }
                      frame True {
                        n219 = call "获取最近两组水样测试数据.vi"("table"="水温") -> ("error out"=w438:errorcluster, "存储变量"=w437:T12)  [unwired: 9 in]
                        n220 = call "集成干预测试数据存储.vi"("error in (no error)"=w438, "存储变量"=w437) -> ("error out"=w435:errorcluster)  [unwired: 9 in]
                      }
                    }
                    n221 = global read "断电保存变量.vi" "pH"() -> (w397:bool)
                    n222 = case shown="真" w397 {
                      tunnel: [_ w431] -> w403
                      tunnel: w404 -> [_ w430]
                      frame False {
                      }
                      frame True {
                        n223 = call "获取最近两组水样测试数据.vi"("error in (no error)"=w430, "table"="pH") -> ("error out"=w434:errorcluster, "存储变量"=w433:T12)  [unwired: 8 in]
                        n224 = call "集成干预测试数据存储.vi"("error in (no error)"=w434, "存储变量"=w433) -> ("error out"=w431:errorcluster)  [unwired: 9 in]
                      }
                    }
                    n225 = global read "断电保存变量.vi" "DO"() -> (w396:bool)
                    n226 = case shown="真" w396 {
                      tunnel: [_ w426] -> w402
                      tunnel: w403 -> [_ w425]
                      frame False {
                      }
                      frame True {
                        n227 = call "获取最近两组水样测试数据.vi"("error in (no error)"=w425, "table"="DO") -> ("error out"=w429:errorcluster, "存储变量"=w428:T12)  [unwired: 8 in]
                        n228 = call "集成干预测试数据存储.vi"("error in (no error)"=w429, "存储变量"=w428) -> ("error out"=w426:errorcluster)  [unwired: 9 in]
                      }
                    }
                    n229 = global read "断电保存变量.vi" "Cond"() -> (w395:bool)
                    n230 = case shown="真" w395 {
                      tunnel: [_ w421] -> w401
                      tunnel: w402 -> [_ w420]
                      frame False {
                      }
                      frame True {
                        n231 = call "获取最近两组水样测试数据.vi"("error in (no error)"=w420, "table"="比电导率") -> ("error out"=w424:errorcluster, "存储变量"=w423:T12)  [unwired: 8 in]
                        n232 = call "集成干预测试数据存储.vi"("error in (no error)"=w424, "存储变量"=w423) -> ("error out"=w421:errorcluster)  [unwired: 9 in]
                      }
                    }
                    n233 = global read "断电保存变量.vi" "Turb"() -> (w394:bool)
                    n234 = case shown="真" w394 {
                      tunnel: [_ w416] -> w400
                      tunnel: w401 -> [_ w415]
                      frame False {
                      }
                      frame True {
                        n235 = call "获取最近两组水样测试数据.vi"("error in (no error)"=w415, "table"="浊度") -> ("error out"=w419:errorcluster, "存储变量"=w418:T12)  [unwired: 8 in]
                        n236 = call "集成干预测试数据存储.vi"("error in (no error)"=w419, "存储变量"=w418) -> ("error out"=w416:errorcluster)  [unwired: 9 in]
                      }
                    }
                    n237 = global read "断电保存变量.vi" "叶绿素a启用"() -> (w393:bool)
                    n238 = case shown="真" w393 {
                      tunnel: [_ w411] -> w399
                      tunnel: w400 -> [_ w410]
                      frame False {
                      }
                      frame True {
                        n239 = call "获取最近两组水样测试数据.vi"("error in (no error)"=w410, "table"="叶绿素") -> ("error out"=w414:errorcluster, "存储变量"=w413:T12)  [unwired: 8 in]
                        n240 = call "集成干预测试数据存储.vi"("error in (no error)"=w414, "存储变量"=w413) -> ("error out"=w411:errorcluster)  [unwired: 9 in]
                      }
                    }
                    n241 = case shown="真" FALSE {
                      tunnel: [_ w406] -> _
                      tunnel: w399 -> [_ w405]
                      frame False {
                      }
                      frame True {
                        n242 = call "获取最近两组水样测试数据.vi"("error in (no error)"=w405, "table"="藻密度") -> ("error out"=w409:errorcluster, "存储变量"=w408:T12)  [unwired: 8 in]
                        n243 = call "集成干预测试数据存储.vi"("error in (no error)"=w409, "存储变量"=w408) -> ("error out"=w406:errorcluster)  [unwired: 9 in]
                      }
                    }
                  }
                }
              }
            }
          }
        }
        n244 = global read "采配水全局变量.vi" "状态"() -> (w293:T8)
        n245 = Unbundle By Name(w293) -> ("R0"=w292:i16)
        n246 = Equal To 0?(x=w292) -> (x = 0?=w291:bool)
        n247 = Select(t=enum16{"初始化", "采配水启动", "仪器操作", "反冲洗", "结束"}."结束" ("枚举"), s=w291, f=enum16{"初始化", "采配水启动", "仪器操作", "反冲洗", "结束"}."反冲洗" ("枚举")) -> (s? t:f=w288:enum16{"初始化", "采配水启动", "仪器操作", "反冲洗", "结束"})
      }
      frame "结束" {
        n248 = Release Queue(queue=w456) -> ()  [unwired: 2 in, 3 out]
        n249 = Unbundle By Name(w453) -> ("测试模式"=w454:enum16{"正常测试", "集成干预"})
        n250 = Cancel Notification(0:w457) -> (8:w458:refnum<notifier>)  [unwired: 1 in, 2 out]
        n251 = Release Notifier(notifier=w458) -> ()  [unwired: 2 in, 3 out]
        n252 = case shown="\"集成干预\"" w454 {
          tunnel: w452 -> [_ w461]
          frame "正常测试", Default {
          }
          frame "集成干预" {
            n253 = global write "系统设置全局变量.vi" "运行模式"(w461) -> ()
          }
        }
      }
    }
    n254 = Format Into String(format string="%s,当前运行时间%d秒" ("格式字符串"), w15, w11) -> (resulting string=w16:string)  [unwired: 2 in, 1 out]
    n255 = global write "采配水全局变量.vi" "运行状态显示"(w16) -> ()
  }
